vi "Display Images Modified.vi"(0 "fpga interface in":refnum<k20>, 1 "'stop' notifier":refnum<notifier>, 2 "rate references":T1, 5 "display channel number":i32, 7 "raw display notifier":refnum<notifier>, 9 "display reference":refnum<vi>, 11 "error in (no error)":errorcluster) -> (4 "fpga interface out":refnum<k20>, 15 "error out":errorcluster)   [LabVIEW 2026, in "GettingStarted_Common_148X_Host.lvlib"]
uses:
  GettingStarted_Common_148X_Host.lvlib
  Types/Serial Channel Display Parameters.ctl
  <vilib>/vision/Image Controls.llb/IMAQ Image.ctl
  Types/RAW Interpretation for Display.ctl
  Types/148x_Common_FPGA_Reference.ctl
  <vilib>/Utility/error.llb/Error Cluster From Error Code.vi
  <vilib>/rvi/errors/niLvFpgaAdjustHostInterfaceError.vi
  <vilib>/rvi/interface/nirviReadWriteControl/nirviReadWriteControl.xnode
  NiFpgaLv.dll
  <vilib>/rvi/interface/Simulation/niFpgaSimulationCallBeginRW.vi
panel:
  out "Display Rate":dbl
  out "Source Rate":dbl
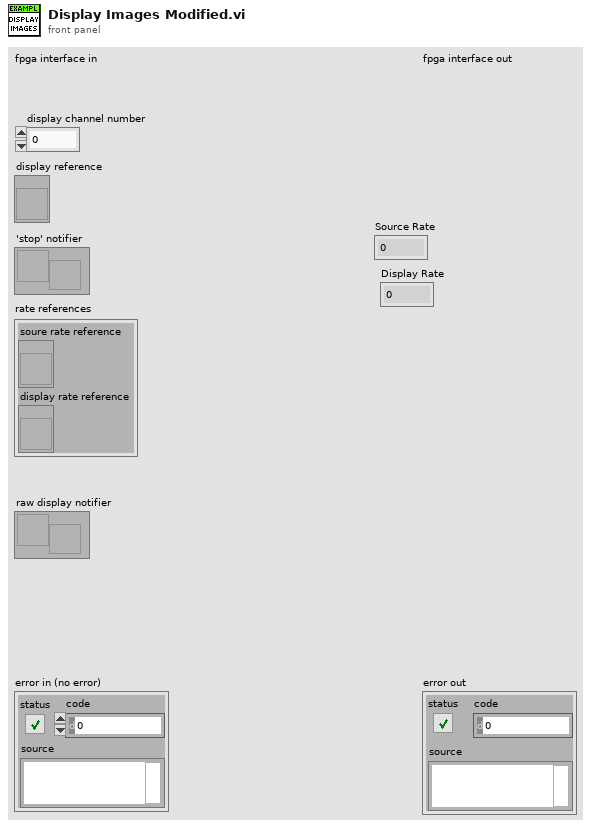
[diagram p1: front panel]
types:
  T1 = cluster{"soure rate reference":refnum<vi>, "display rate reference":refnum<vi>}
  T2 = typedef "GettingStarted_Common_148X_Host.lvlib/148x_Common_FPGA_Reference.ctl" = refnum<k20>
  T3 = typedef "GettingStarted_Common_148X_Host.lvlib/Serial Channel Display Parameters.ctl" = cluster{"images":cluster{"grayscale":T4, "color":T4}, "RAW parameters":cluster{"interpretation":T5, "bayer parameters":cluster{"pattern":i32, "algorithm":i32, "red gain":dbl, "green gain":dbl, "blue gain":dbl}}}
  T4 = typedef "IMAQ Image.ctl" = refnum<image>
  T5 = typedef "GettingStarted_Common_148X_Host.lvlib/RAW Interpretation for Display.ctl" = enum16{"Grayscale", "Bayer", "RGB", "YUV422", "YUV420", "Legacy YUV420"}
  T6 = typedef "GettingStarted_Common_148X_FPGA.lvlib/Image Metadata.ctl" = cluster{"serial channel":fxp<+,3,3>, "frame number":u16, "data type":T7, "width":u16, "height":u16, "image bytes":u32, "total bytes":u32, "little endian":bool}
  T7 = typedef "NI CSI-2 API Common v2.lvlib/LLP Data Type.ctl" = enum8{"Frame Start", "Frame End", "Line Start", "Line End", "End of Transmission", "Reserved 0", "Reserved 1", "Reserved 2", "Generic Short Packet 1", "Generic Short Packet 2", "Generic Short Packet 3", "Generic Short Packet 4", "Generic Short Packet 5", "Generic Short Packet 6", "Generic Short Packet 7", "Generic Short Packet 8", "Null", "Blanking Data", "Embedded 8-bit non Image Data", "Generic Long Packet 1", "Generic Long Packet 2", "Generic Long Packet 3", "Generic Long Packet 4", "Reserved 3", "YUV420 8-bit", "YUV420 10-bit", "Legacy YUV420 8-bit", "Reserved 4", "YUV420 8-bit Chroma Shifted", "YUV420 10-bit Chroma Shifted", "YUV422 8-bit", "YUV422 10-bit", "RGB444", "RGB555", "RGB565", "RGB666", "RGB888", "Reserved 5", "Reserved 6", "RAW 24", "RAW 6", "RAW 7", "RAW 8", "RAW 10", "RAW 12", "RAW 14", "RAW 16", "RAW 20", "User Defined 8-bit Data 1", "User Defined 8-bit Data 2", "User Defined 8-bit Data 3", "User Defined 8-bit Data 4", "User Defined 8-bit Data 5", "User Defined 8-bit Data 6", "User Defined 8-bit Data 7", "User Defined 8-bit Data 8", "USL Command", "Reserved 7", "Reserved 8", "Reserved 9", "Reserved 10", "Reserved 11", "Reserved 12", "LRTE EPD Spacer"}
  T8 = cluster{"image pixel data fifo overflow":bool, "image metadata fifo overflow":bool}[]
  T9 = cluster{"image pixel data fifo overflow":bool, "image metadata fifo overflow":bool}
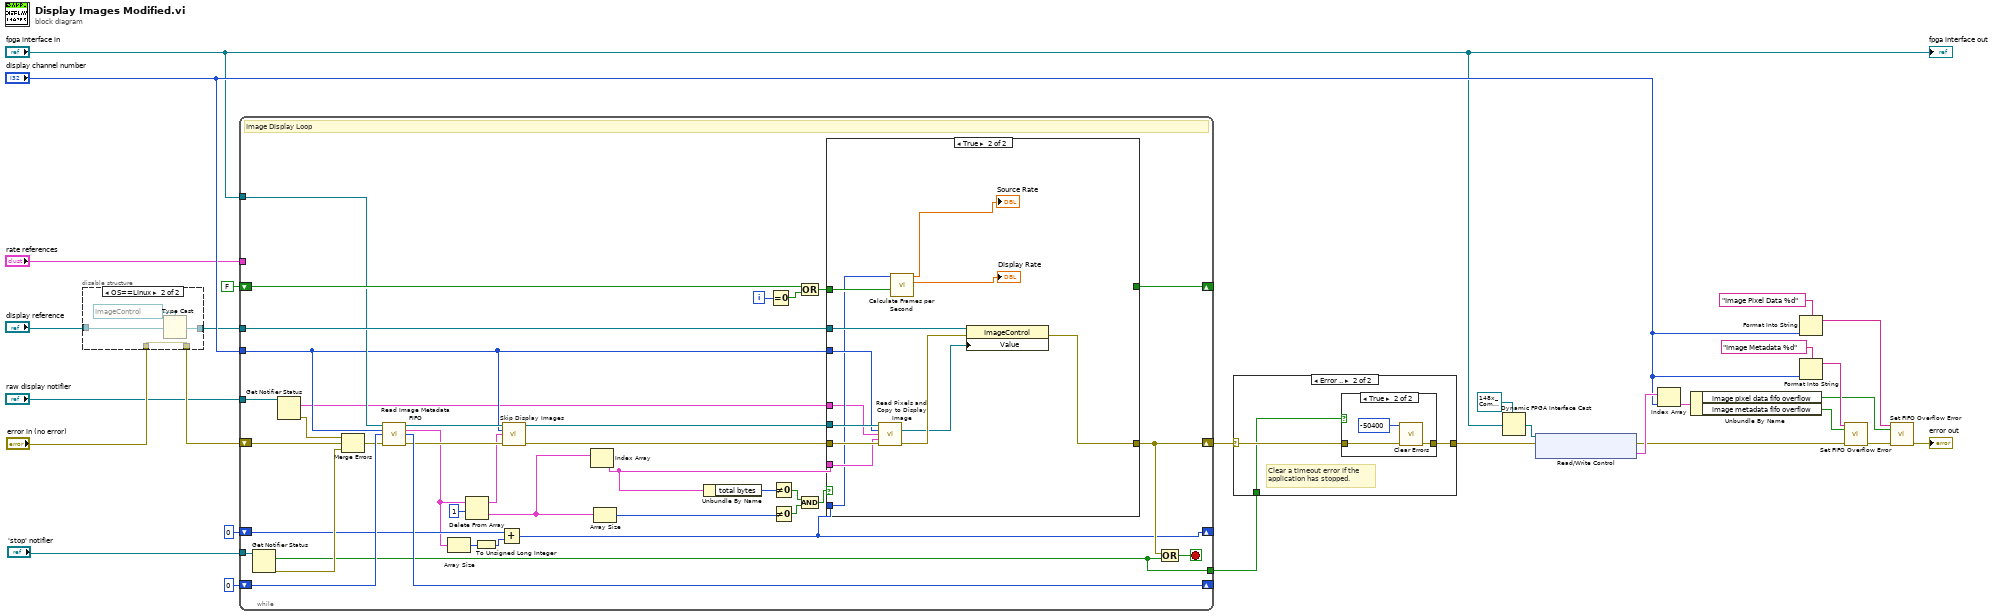
[diagram p0: block diagram]
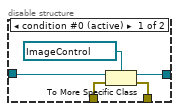
[diagram p2: hidden frame]
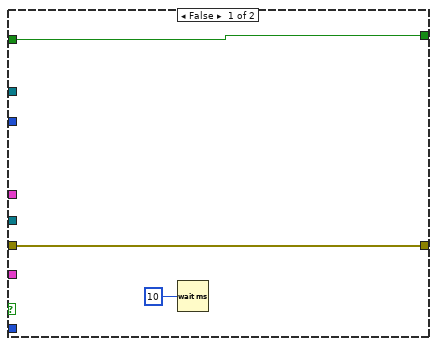
[diagram p3: hidden frame]
diagram:
  n1 = disable-structure shown="OS==Linux" {
    disable-tunnel: "display reference" -> [w32 w35]
    disable-tunnel: "error in (no error)" -> [w29 w36]
    disable-tunnel: [w31 w34] -> w5
    disable-tunnel: [w30 w36] -> w4
    frame condition #0 (active) {
      n2 = To More Specific Class(target class=refnum<vi> refnum ("reference"), reference=w32, error in=w29) -> (specific class reference=w31:refnum<vi>, error out=w30:errorcluster)
    }
    frame condition #1 {
      n3 = Type Cast(type=refnum<vi> refnum ("reference"), x=w35) -> (*(type *) &x=w34:refnum<vi>)
    }
  }
  n4 = while {
    shift-right: [w72] -> w9
    shift-left: w4 -> [w42]
    tunnel: "fpga interface in" -> [w46]
    shift-right: [w73] -> _
    shift-left: u32 0 ("Elements Remaining") -> [w60]
    tunnel: "display channel number" -> [w41]
    tunnel: w5 -> [w71]
    tunnel: "rate references" -> [_]
    shift-right: [w64] -> _
    shift-left: FALSE -> [w61]
    shift-right: [w48] -> _
    shift-left: u32 0 ("Elements Remaining") -> [w51]
    tunnel: [w44] -> w3
    tunnel: "'stop' notifier" -> [w45]
    tunnel: "raw display notifier" -> [w40]
    i -> [w70]
    stop <- w74 stop-if-true
    # "Image Display Loop"
    n5 = Get Notifier Status(notifier=w45) -> (current notification=w44:bool, error out=w75:errorcluster)  [unwired: 1 in, 3 out]
    n6 = Get Notifier Status(notifier=w40) -> (current notification=w39:T3[], error out=w38:errorcluster)  [unwired: 1 in, 3 out]
    n7 = Merge Errors(w38, w42, w75) -> (w43:errorcluster)
    n8 = call "Read Image Metadata FIFO.vi"("fpga inteface in"=w46, "display channel number"=w41, "number of images"=w60, "error in (no error)"=w43) -> ("fpga interface out"=w56:refnum<k20>, "image metadata"=w47:T6[], "images remaining"=w73:u32, "error out"=w53:errorcluster)  [unwired: 8 in]
    n9 = Array Size(array=w47) -> (size(s)=w50:i32)
    n10 = Delete From Array(array=w47, length=1) -> (deleted portion=w57:T6[], array with subset deleted=w52:T6[])  [unwired: 1 in]
    n11 = To Unsigned Long Integer(number=w50) -> (unsigned 32bit integer=w49:u32)
    n12 = Add(x=w51, y=w49) -> (x+y=w48:u32)
    n13 = call "Skip Display Images.vi"("fpga interface in"=w56, "display channel number"=w41, "image metadata"=w52, "error in (no error)"=w53) -> ("fpga interface out"=w55:refnum<k20>, "error out"=w54:errorcluster)  [unwired: 10 in]
    n14 = Index Array(array=w57) -> (element=w69:T6)  [unwired: 1 in]
    n15 = Array Size(array=w57) -> (size(s)=w59:i32)
    n16 = Unbundle By Name(w69) -> ("total bytes"=w68:u32)
    n17 = Equal To 0?(x=w70) -> (x = 0?=w62:bool)
    n18 = Not Equal To 0?(x=w68) -> (x != 0?=w66:bool)
    n19 = Not Equal To 0?(x=w59) -> (x != 0?=w67:bool)
    n20 = Compound Arithmetic op=OR(w61, w62) -> (w63:bool)
    n21 = Compound Arithmetic op=AND(w66, w67) -> (w65:bool)
    n22 = case shown="True" w65 {
      tunnel: w54 -> [w78 w91]
      tunnel: w55 -> [_ w90]
      tunnel: w39 -> [_ w81]
      tunnel: w41 -> [_ w89]
      tunnel: [w78 w88] -> w72
      tunnel: w71 -> [_ w87]
      tunnel: w69 -> [_ w86]
      tunnel: w63 -> [w76 w85]
      tunnel: [w76 _] -> w64
      tunnel: w48 -> [_ w84]
      frame False {
        n23 = Wait (ms)(milliseconds to wait=u32 10) -> ()  [unwired: 1 out]
      }
      frame True {
        n24 = call "Read Pixels and Copy to Display Image.vi"("fpga interface in"=w90, "display channel number"=w89, "serial channel display parameters"=w81, "image metadata"=w86, "error in (no error)"=w91) -> ("display image"=w82:T4, "error out"=w83:errorcluster)  [unwired: 8 in, 1 out]
        n25 = call <vilib>:"Calculate Frames per Second.vi"("Reset"=w85, "Buffer Number"=w84) -> ("Processed Frames/s"=→"Display Rate":dbl, "Acquired Frames/s"=→"Source Rate":dbl)  [unwired: 7 in, 1 out]
        n26 = property class="ImageControl"(reference=w87, error in=w83, "Value"=w82) -> (error out=w88:errorcluster)  [unwired: 1 out]
      }
    }
    n27 = Compound Arithmetic op=OR(w72, w44) -> (w74:bool)
  }
  n28 = case shown="Error .." w9 {
    selector: w9 -> [w92 w95]
    tunnel: [w92 w94] -> w23
    tunnel: w3 -> [_ w93]
    frame No Error {
    }
    frame Error {
      # "Clear a timeout error if the application has stopped."
      n29 = case shown="True" w93 {
        tunnel: w95 -> [w96 w99]
        tunnel: [w96 w97] -> w94
        frame False {
        }
        frame True {
          n30 = call <vilib>:"Clear Errors.vi"("error in (no error)"=w99, "specific error code to clear (0: all)"=-50400 ("y")) -> ("error out"=w97:errorcluster)  [unwired: 4 in, 1 out]
        }
      }
    }
  }
  n31 = Dynamic FPGA Interface Cast(Session In=T2 refnum ("FPGA VI Reference Out"), Type="fpga interface in") -> (Session Out=w24:T2)
  n32 = xnode "Read/Write Control"("FPGA VI Reference In"=w24, "error in"=w23) -> ("error out"=w22:errorcluster, "display channel status"=w26:T8)  [unwired: 1 out]
  n33 = Index Array(array=w26, index="display channel number") -> (element=w27:T9)
  n34 = Unbundle By Name(w27) -> ("image pixel data fifo overflow"=w14:bool, "image metadata fifo overflow"=w13:bool)
  n35 = Format Into String(format string="Image Pixel Data %d", "display channel number") -> (resulting string=w16:string)  [unwired: 2 in, 1 out]
  n36 = Format Into String(format string="Image Metadata %d", "display channel number") -> (resulting string=w15:string)  [unwired: 2 in, 1 out]
  n37 = call "Set FIFO Overflow Error.vi"("fifo name"=w15, "overflow"=w13, "error in (no error)"=w22) -> ("error out"=w18:errorcluster)  [unwired: 12 in]
  n38 = call "Set FIFO Overflow Error.vi"("fifo name"=w16, "overflow"=w14, "error in (no error)"=w18) -> ("error out"=→"error out":errorcluster)  [unwired: 12 in]
  "fpga interface out" <- "fpga interface in"
